vi "array.vi"() -> ()   [LabVIEW 2019]
panel:
  out "element 3":bool
  in  "index 2":i32
  in  "Array 3":bool[](array[boolean])
  out "element 2":dbl
  in  "disabled index (col)":i32
  out "subarray":dbl[](array[numeric])
  in  "Array 2":dbl[][](array[numeric])
  out "element":dbl
  in  "index":i32
  in  "Array":dbl[](array[numeric])
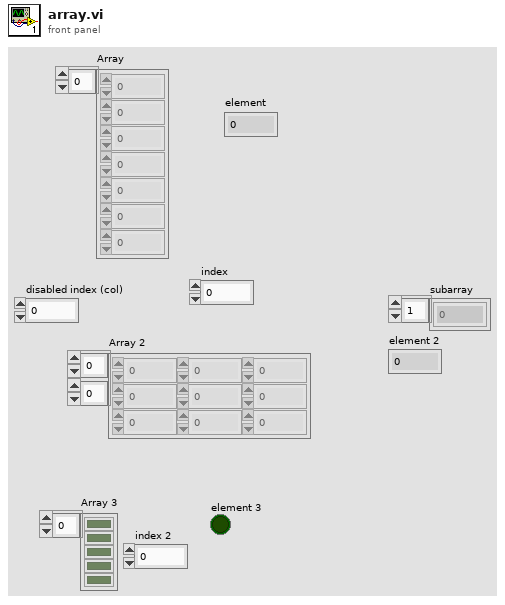
[diagram p1: front panel]
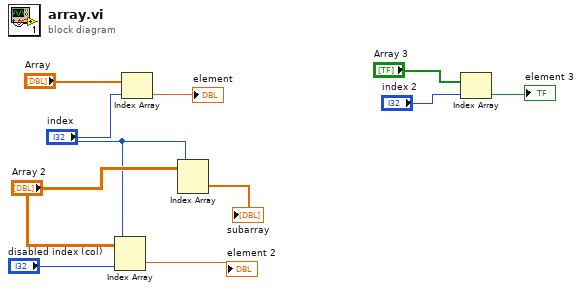
[diagram p0: block diagram]
diagram:
  n1 = Index Array(array="Array 2", index (row)="index", index (col)="disabled index (col)") -> (element=→"element 2":dbl)
  n2 = Index Array(array="Array", index="index") -> (element=→"element":dbl)
  n3 = Index Array(array="Array 2", index (row)="index") -> (element=→"subarray":dbl[])  [unwired: 1 in]
  n4 = Index Array(array="Array 3", index="index 2") -> (element=→"element 3":bool)
